vi "Record Auto Restart.vi"(8 "error in (no error)":errorcluster, 10 "Automatically restart acquisition on end?":bool, 11 "VISA resource name":refnum<visa-resource-name>) -> (0 "error out":errorcluster, 3 "VISA resource name out":refnum<visa-resource-name>)   [LabVIEW 2017, in "Sefram DAS220.lvlib"]
doc: "Set the record automatically restart after records end."
uses:
  <instrlib>/Sefram DAS220/Sefram DAS220.lvlib
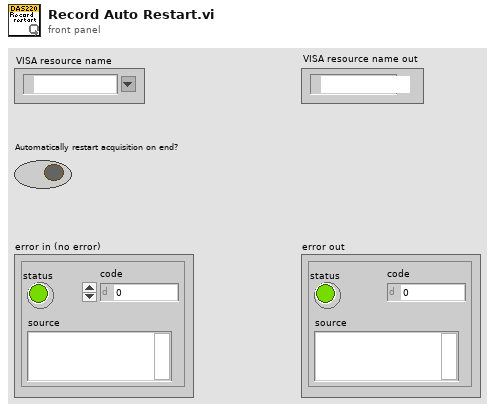
[diagram p1: front panel]
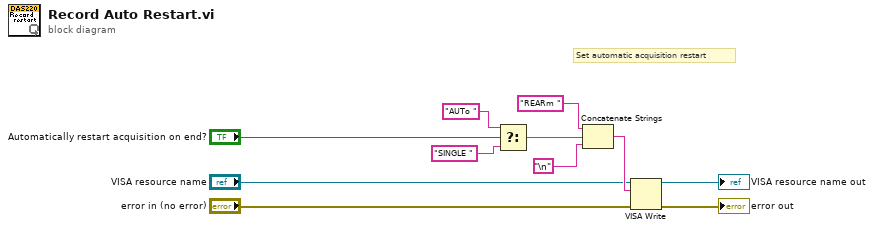
[diagram p0: block diagram]
diagram:
  # "Set automatic acquisition restart"
  n1 = Select(t="AUTo " ("string"), s="Automatically restart acquisition on end?", f="SINGLE " ("string")) -> (s? t:f=w1:string)
  n2 = Concatenate Strings("REARm " ("string"), w1, "\n") -> (w11:string)
  n3 = VISA Write(VISA resource name="VISA resource name", write buffer=w11, error in (no error)="error in (no error)") -> (VISA resource name out=→"VISA resource name out":refnum<visa-resource-name>, error out=→"error out":errorcluster)  [unwired: 1 out]
